vi "Scale Waveform.vi"(8 "Error In":errorcluster, 9 "Read Size":i32, 11 "Async State Vars 2":T1) -> (0 "Error Out":errorcluster, 3 "Async State Vars out":T1)   [LabVIEW 2020, in "Waveform-Processing-Custom-Device Shared.lvlib" / "Scaled Waveform.lvlib"]
uses:
  Shared/Scaled Waveform/Scaled Waveform.lvlib
  <userlib>/Circular Buffer/Controls/Circular Buffer Operations.ctl
  <vilib>/NI/NIVS Inline Async API/_Data Access Engine/Data Access Engine/Data Access Engine.lvclass
  <vilib>/NI/NIVS Inline Async API/_Data Access Engine/Data Access Engine/Methods/Read.Data.vi
  <userlib>/Circular Buffer/Instance VIs/Circular Buffer(2D DBL).vi
  <vilib>/NI VeriStand/Custom Device Waveform API/Single Waveform Read (DBL)/Single Waveform Read (DBL).lvclass
  Types/AsyncStateVariables.ctl
  Waveform-Processing-Custom-Device Engine.lvlib
  <vilib>/NI VeriStand/Custom Device Waveform API/Single Waveform Write (DBL)/Single Waveform Write (DBL).lvclass
  <vilib>/NI VeriStand/Custom Device API/Waveform Data Reference.ctl
  <vilib>/NI VeriStand/Custom Device API/Custom Device API.lvlib
  <vilib>/NI/NIVS Inline Async API/_Data Access Engine/Access Type Classes/Read/Read.lvclass
  <vilib>/NI/NIVS Inline Async API/_Data Access Engine/Data Access Engine/Types/Read.DVR.ctl
  <vilib>/NI/NIVS Inline Async API/_Data Access Engine/Access Type Classes/Write/Write.lvclass
  <vilib>/NI/NIVS Inline Async API/_Data Access Engine/Data Access Engine/Types/Write.DVR.ctl
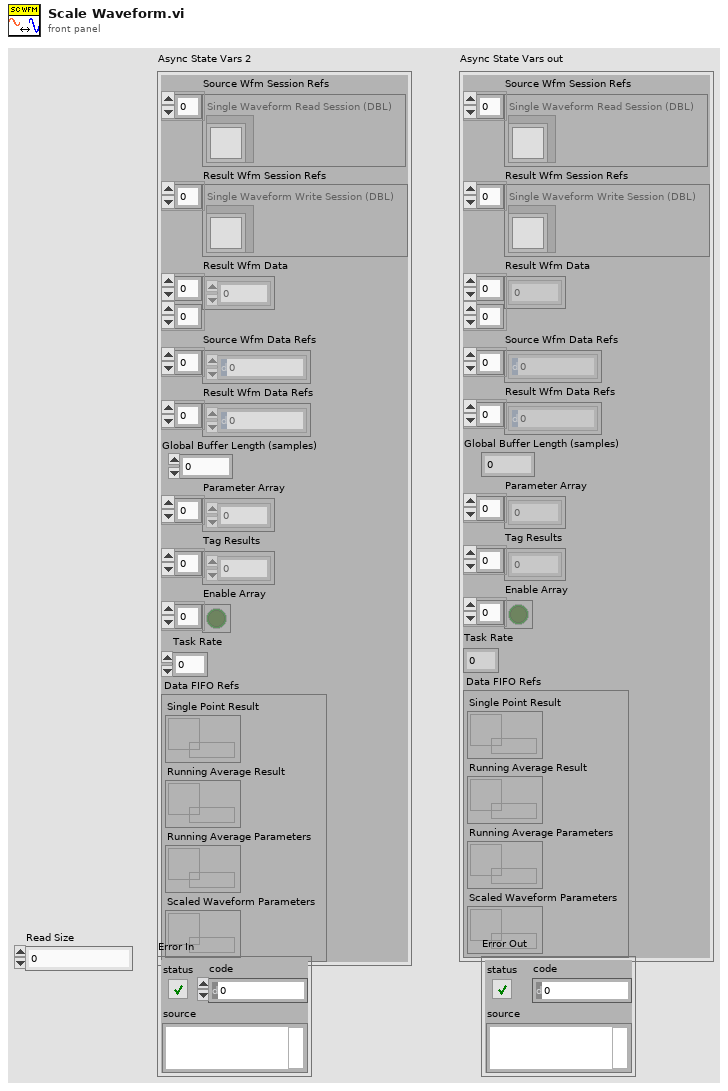
[diagram p1: front panel]
types:
  T1 = typedef "Waveform-Processing-Custom-Device Engine.lvlib/AsyncStateVariables.ctl" = cluster{"Source Wfm Session Refs":refnum<class "Single Waveform Read (DBL).lvclass">[], "Result Wfm Session Refs":refnum<class "Single Waveform Write (DBL).lvclass">[], "Result Wfm Data":dbl[][], "Source Wfm Data Refs":T2[], "Result Wfm Data Refs":T2[], "Global Buffer Length (samples)":dbl, "Parameter Array":dbl[], "Tag Results":dbl[], "Enable Array":bool[], "Task Rate":dbl, "Data FIFO Refs":cluster{"Single Point Result":T3, "Running Average Result":T3, "Running Average Parameters":T4, "Scaled Waveform Parameters":T4}}
  T2 = typedef "Custom Device API.lvlib/Waveform Data Reference.ctl" = i32
  T3 = typedef "Data Access Engine.lvlib/Data Access Engine.lvclass/Write.DVR.ctl" = refnum<data-value>
  T4 = typedef "Data Access Engine.lvlib/Data Access Engine.lvclass/Read.DVR.ctl" = refnum<data-value>
  T5 = typedef "Circular Buffer.lvlib/Circular Buffer Operations.ctl" = enum16{"Initialize", "Get Backlog", "Write", "Read (continuous)", "Read (most recent)"}
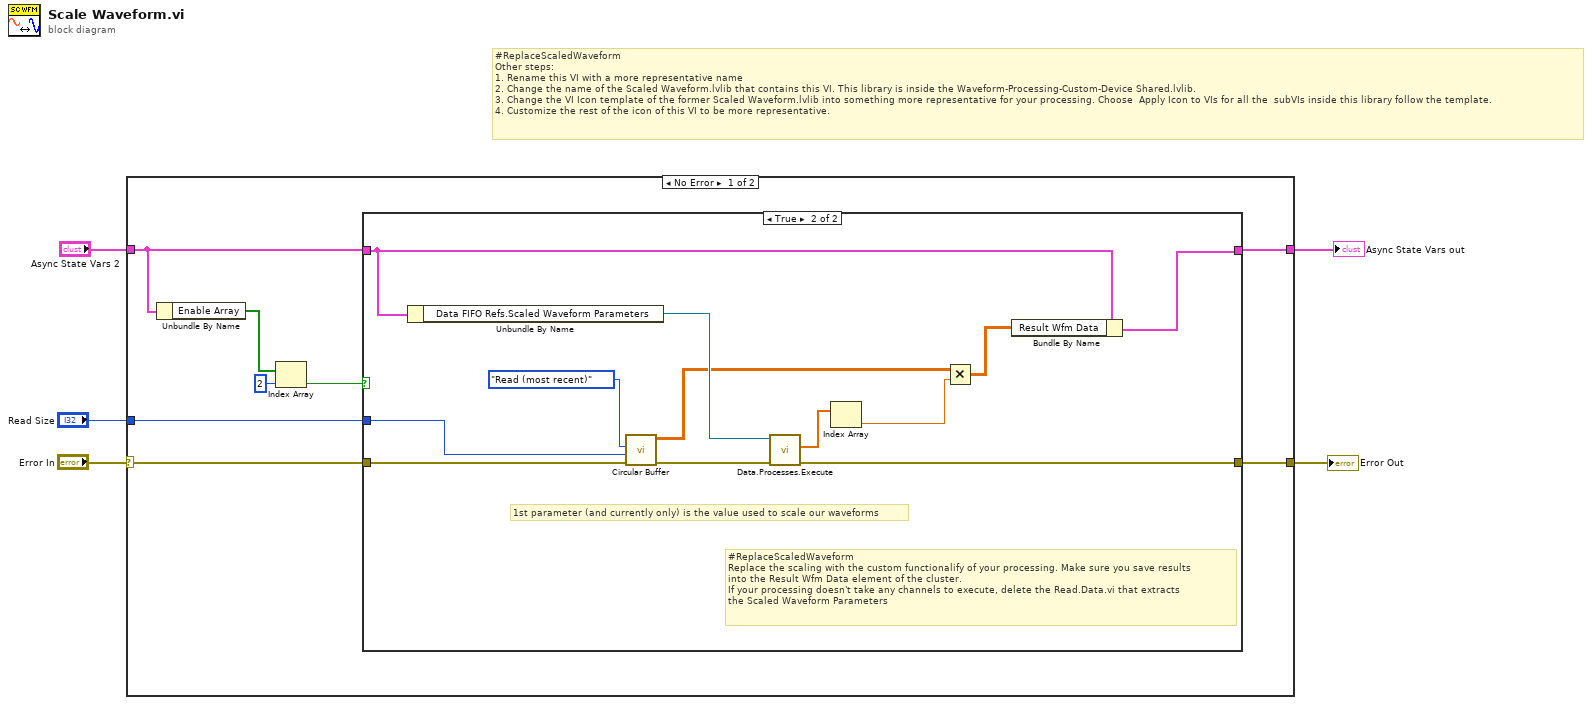
[diagram p0: block diagram]
diagram:
  # "#ReplaceScaledWaveform \nOther steps:\n1. Rename this VI with a more representative name\n2. Change the name of the Scaled Waveform.lvlib that contains this VI. This library is inside the Waveform-Processing-Custom-Device Shared.lvlib.\n3. Change the VI Icon template of the former Scaled Waveform.lvlib into something more representative for your processing. Choose  Apply Icon to VIs for all the  subVIs inside this library follow the template.\n4. Customize the rest of the icon of this VI to be more representative."
  n1 = case shown="No Error" "Error In" {
    selector: "Error In" -> [w13 w29]
    tunnel: [w12 w29] -> w4
    tunnel: "Async State Vars 2" -> [w10 w28]
    tunnel: [w11 w28] -> w2
    tunnel: "Read Size" -> [w6 _]
    frame No Error {
      n2 = Unbundle By Name(w10) -> ("Enable Array"=w9:bool[])
      n3 = Index Array(array=w9, index=2) -> (element=w8:bool)
      n4 = case shown="True" w8 {
        tunnel: w13 -> [w15 w26]
        tunnel: [w15 w16] -> w12
        tunnel: w10 -> [w14 w21]
        tunnel: [w14 w17] -> w11
        tunnel: w6 -> [_ w25]
        frame False {
        }
        frame True {
          # "#ReplaceScaledWaveform \nReplace the scaling with the custom functionalify of your processing. Make sure you save results\ninto the Result Wfm Data element of the cluster.\nIf your processing doesn't take any channels to execute, delete the Read.Data.vi that extracts\nthe Scaled Waveform Parameters"
          # "1st parameter (and currently only) is the value used to scale our waveforms"
          n5 = Unbundle By Name(w21) -> ("Data FIFO Refs.Scaled Waveform Parameters"=w22:T4)
          n6 = call-poly <userlib>:"Circular Buffer.vi"("error in (no error)"=w26, "Read Size"=w25, "Operation"=Circular_Buffer_Operations."Read (most recent)") -> ("error out"=w23:errorcluster, "Data Out"=w20:dbl[][])  [unwired: 5 in, 2 out]
          n7 = call-poly <vilib>:"Data.Processes.Execute.vi"("error in (no error)"=w23, "Ref"=w22) -> ("error out"=w16:errorcluster, "Values"=w24:dbl[])  [unwired: 7 in, 1 out]
          n8 = Index Array(array=w24) -> (element=w19:dbl)  [unwired: 1 in]
          n9 = Multiply(x=w20, y=w19) -> (x*y=w18:dbl[][])
          n10 = Bundle By Name(cluster=w21, "Result Wfm Data"=w18) -> (w17:T1)
        }
      }
    }
    frame Error {
    }
  }
  "Error Out" <- w4
  "Async State Vars out" <- w2
